vi "SyringeCalibration.vi"() -> ()   [LabVIEW 2019]
panel:
  out "ValidZ?":bool
  out "ValidY?":bool
  out "ValidX?":bool
  out "FinalXYZ":string
  in  "ExtraKaptonZ(mm)":dbl
  in  "HeightGaugeOffset(mm)":dbl=50.5
  out "CorrPosZ":dbl
  out "error out":errorcluster
  out "CorrPosY":dbl
  out "CorrPosX":dbl
  in  "BasePlatePositions":path=path "C:/Users/TTUHEP/Documents/LabVIEW/Data/AssemblyIO_logs/BaseplatePositions.txt"
  in  "RefSyringeYonTray":dbl=1216.51
  in  "RefSyringeXonTray":dbl=487.35
  in  "GHtoSyringeOffsetY":dbl=9.003
  in  "GHtoSyringeOffsetX":dbl=135.44
  in  "OnBaseplate":bool
  in  "ZcalibGcodeOnBaseplate":string="G90\nG1 Z0 F100\nG1 X368.574\tY1136.68\tF100\nG1 Z25.988 F10"
  out "TouchStatusY":bool
  out "TouchOnceY?":bool
  out "TouchStatusX":bool
  in  "StopX":bool
  out "TouchOnceX?":bool
  out "TouchedOnce?":bool
  out "TouchStatus":bool
  in  "CalibZ":bool
  in  "CalibY":bool
  in  "CalibX":bool
  out "Position Z":dbl
  in  "StopZ":bool
  out "PositionTrayY":dbl
  in  "StopY":bool
  out "PositionTrayX":dbl
  in  "milliseconds to wait":u32=500
  in  "ZcalibGcode":string="G90\nG1 Z0 F100\nG1 X290.667\tY775.823\tF100\nG1 Z36.5 F10"
  in  "YcalibGcode":string="G90\nG1 Z0 F100\nG1 X450.0 Y1217.0 F100\nG1 Z88.580 F10"
  in  "XcalibGcode":string="G90\nG1 Z0 F100\nG1 X487.5 Y1190.0 F100\nG1 Z88.580 F10"
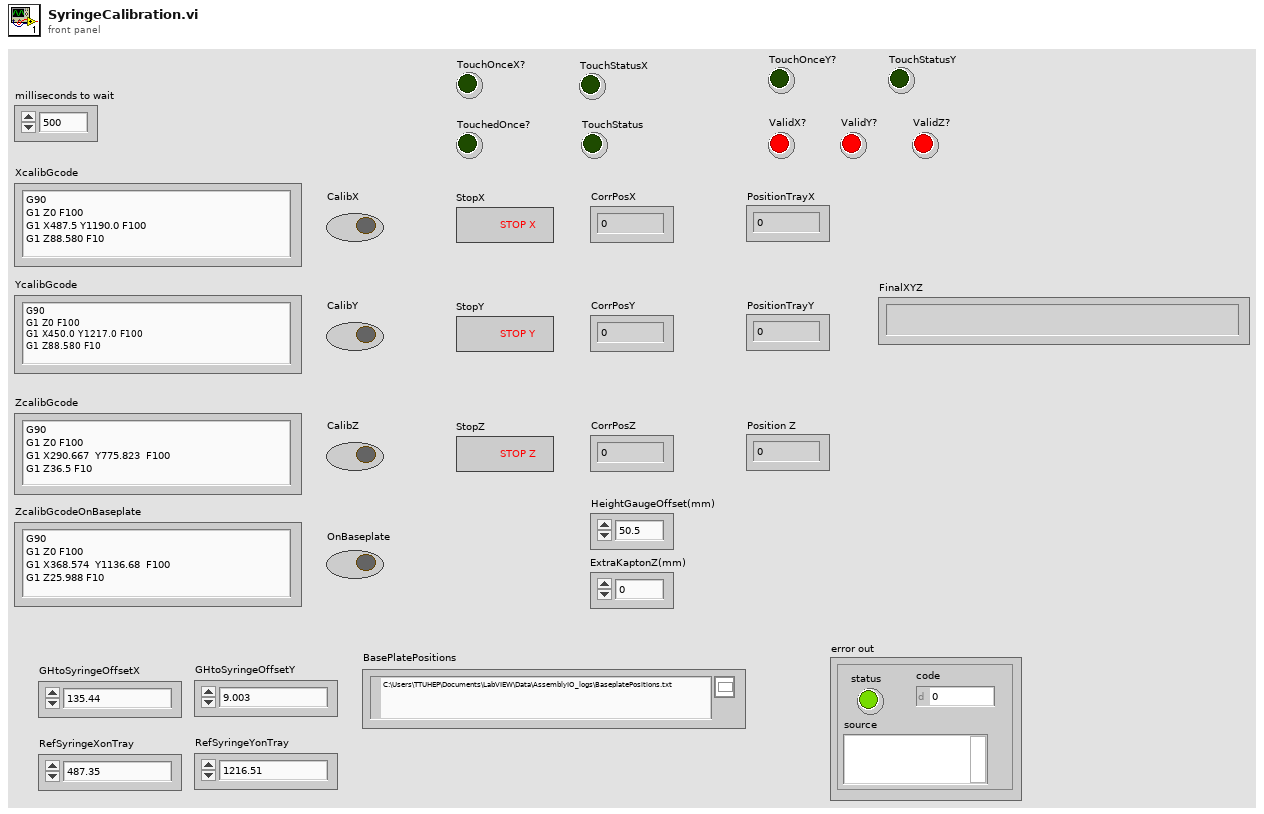
[diagram p1: front panel]
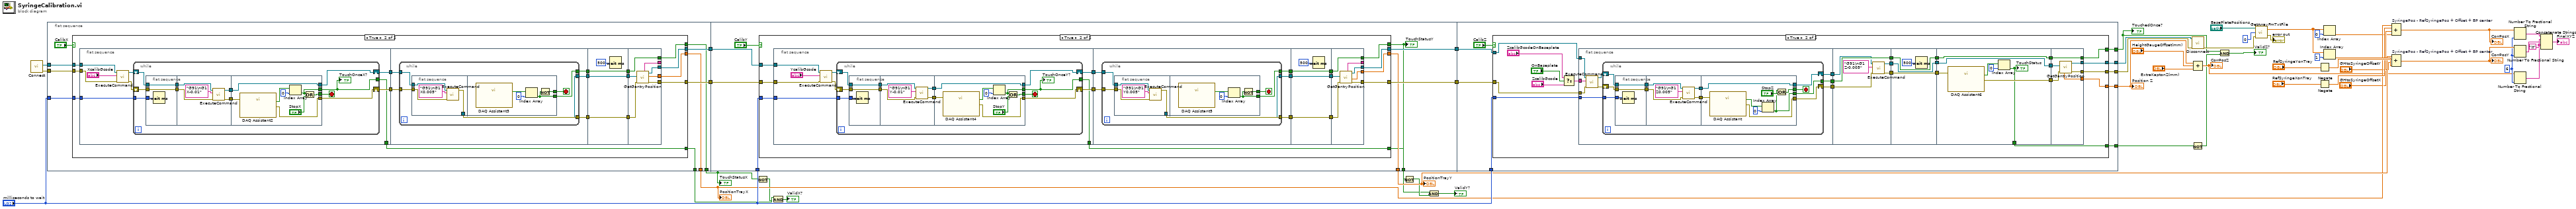
[diagram p0: block diagram]
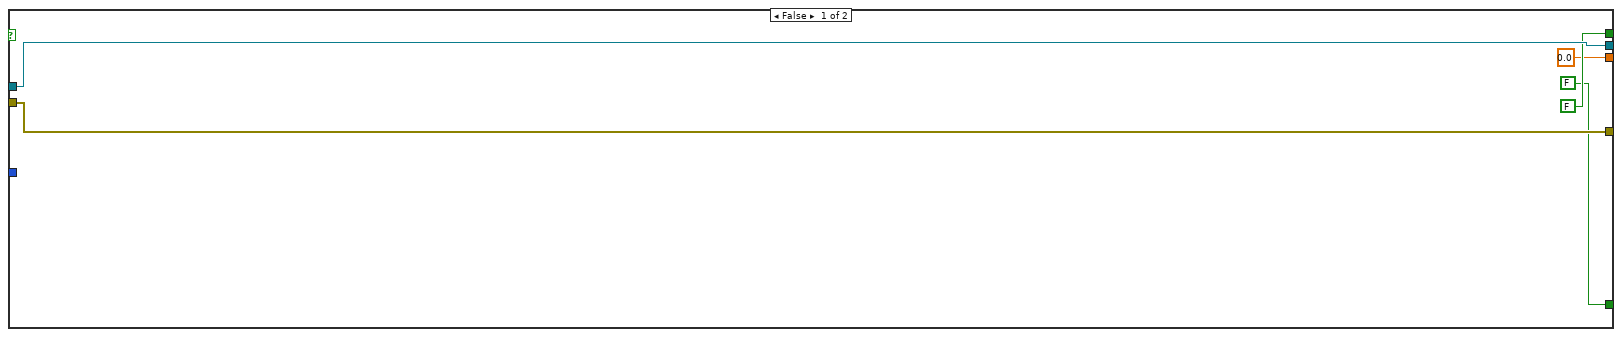
[diagram p2: hidden frame]
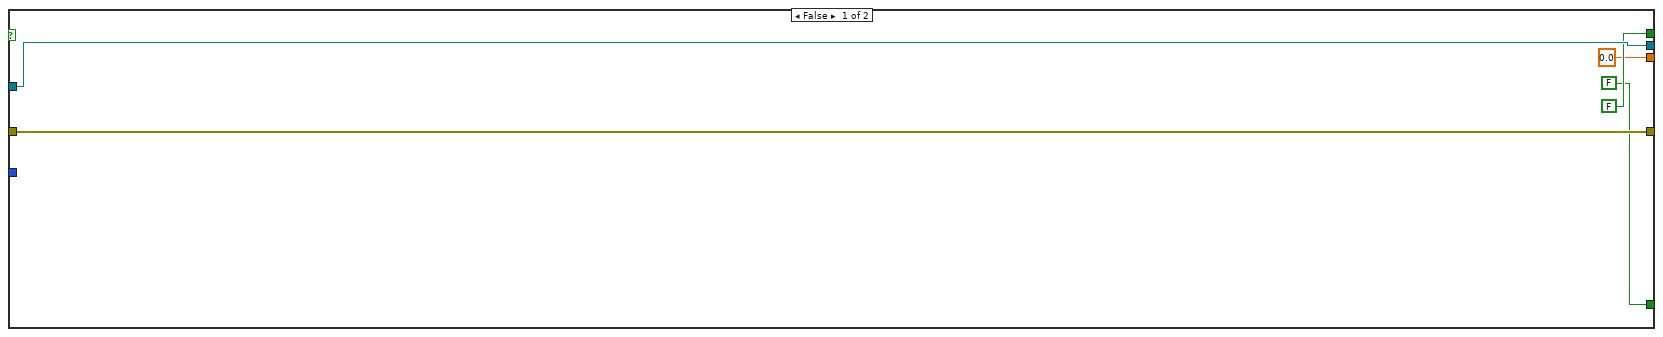
[diagram p3: hidden frame]
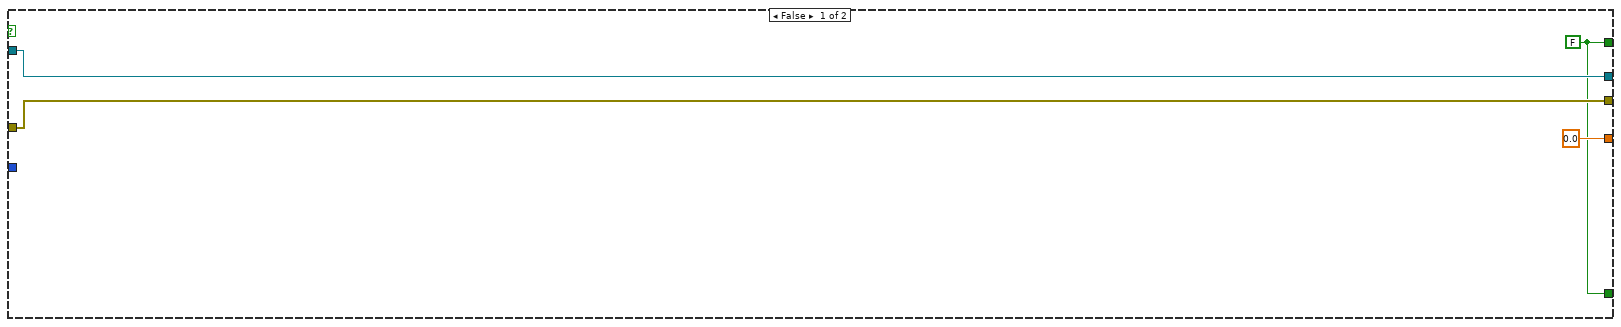
[diagram p4: hidden frame]
diagram:
  w17 = "\t"
  w19 = i16 6 ("width (-)")
  n1 = call "Connect.vi"() -> ("error out"=w47:errorcluster, "controller"=w46:refnum<k24>)  [unwired: 10 in]
  n2 = flat-sequence {
    tunnel: "milliseconds to wait" -> [w56]
    tunnel: w47 -> [w57]
    tunnel: w46 -> [w58]
    tunnel: [w55] -> w45
    tunnel: [w54] -> w44
    tunnel: [w53] -> w10
    tunnel: [w52] -> w31
    tunnel: [w51] -> w12
    tunnel: "milliseconds to wait" -> [w154]
    tunnel: w45 -> [w156]
    tunnel: w44 -> [w155]
    tunnel: [w153] -> w43
    tunnel: [w152] -> w42
    tunnel: [w150] -> w33
    tunnel: [w149] -> w6
    tunnel: [w148] -> w5
    tunnel: "milliseconds to wait" -> [w253]
    tunnel: [w252] -> w49
    tunnel: [w251] -> w48
    tunnel: w43 -> [w249]
    tunnel: [w247] -> w2
    tunnel: w42 -> [w248]
    tunnel: [w246] -> w22
    tunnel: [w245] -> w1
    frame #0 {
      n3 = case shown="True" "CalibX" {
        tunnel: w56 -> [_ w80]
        tunnel: [w64 w74] -> w54
        tunnel: [w63 w73] -> w55
        tunnel: w57 -> [w64 w78]
        tunnel: w58 -> [w63 w79]
        tunnel: [FALSE ("Boolean") w77] -> w53
        tunnel: [0.0 ("Position X") w66] -> w52
        tunnel: [FALSE ("Boolean") w65] -> w51
        frame False {
        }
        frame True {
          n4 = flat-sequence {
            tunnel: w80 -> [w89]
            tunnel: w79 -> [w86]
            tunnel: w78 -> [w85]
            tunnel: [w83] -> w76
            tunnel: [w82] -> w75
            tunnel: [w81] -> w65
            tunnel: w76 -> [w121]
            tunnel: w75 -> [w120]
            tunnel: [w117] -> w72
            tunnel: [w119] -> w70
            tunnel: [w118] -> w68
            tunnel: w72 -> [w140]
            tunnel: [w140] -> w71
            tunnel: w70 -> [w139]
            tunnel: [w139] -> w69
            tunnel: w68 -> [w138]
            tunnel: [w138] -> w67
            tunnel: [w147] -> w77
            tunnel: w71 -> [w147]
            tunnel: w69 -> [w146]
            tunnel: w67 -> [w145]
            tunnel: [w144] -> w74
            tunnel: [w143] -> w73
            tunnel: [w142] -> _
            tunnel: [w141] -> w66
            frame #0 {
              n5 = call "ExecuteCommand.vi"("error in (no error)"=w85, "Command Code"="XcalibGcode", "controller in"=w86) -> ("error out"=w88:errorcluster, "controller out"=w87:refnum<k24>)  [unwired: 6 in, 1 out]
              n6 = while {
                tunnel: w89 -> [w91]
                shift-right: [w96] -> w82
                shift-left: w87 -> [w100]
                shift-right: [w95] -> w83
                shift-left: w88 -> [w99]
                tunnel: [w90] -> w81
                stop <- w94 stop-if-true
                n7 = flat-sequence {
                  tunnel: w99 -> [w102]
                  tunnel: w100 -> [w103]
                  tunnel: [w103] -> w93
                  tunnel: [w102] -> w92
                  tunnel: w91 -> [w101]
                  tunnel: [w105] -> w98
                  tunnel: [w104] -> w97
                  tunnel: w93 -> [w107]
                  tunnel: w92 -> [w106]
                  tunnel: [w111] -> w95
                  tunnel: w98 -> [w112]
                  tunnel: [w116] -> w96
                  tunnel: w97 -> [w116]
                  tunnel: [w113] -> w94
                  tunnel: [w110] -> w90
                  frame #0 {
                    n8 = Wait (ms)(milliseconds to wait=w101) -> ()  [unwired: 1 out]
                  }
                  frame #1 {
                    n9 = call "ExecuteCommand.vi"("error in (no error)"=w106, "Command Code"="G91\nG1 X-0.01", "controller in"=w107) -> ("error out"=w105:errorcluster, "controller out"=w104:refnum<k24>)  [unwired: 6 in, 1 out]
                  }
                  frame #2 {
                    n10 = call "DAQ Assistant2"("error in"=w112) -> ("data"=w114:bool[], "error out"=w111:errorcluster)  [unwired: 16 in, 1 out]
                    n11 = Index Array(array=w114, index=0) -> (element=w110:bool)
                    n12 = Or(x=w110, y="StopX") -> (x .or. y?=w113:bool)
                  }
                }
                "TouchOnceX?" <- w90
              }
            }
            frame #1 {
              n13 = while {
                tunnel: w121 -> [w127]
                tunnel: w120 -> [w126]
                tunnel: [w125] -> w119
                tunnel: [w124] -> w118
                tunnel: [w122] -> w117
                stop <- w123 stop-if-true
                n14 = flat-sequence {
                  tunnel: w127 -> [w132]
                  tunnel: w126 -> [w130]
                  tunnel: [w129] -> w125
                  tunnel: [w128] -> w124
                  tunnel: [w134] -> w123
                  tunnel: [w133] -> w122
                  frame #0 {
                    n15 = call "ExecuteCommand.vi"("error in (no error)"=w132, "Command Code"="G91\nG1 X0.005", "controller in"=w130) -> ("error out"=w129:errorcluster, "controller out"=w128:refnum<k24>)  [unwired: 6 in, 1 out]
                  }
                  frame #1 {
                    n16 = call "DAQ Assistant3"() -> ("data"=w136:bool[])  [unwired: 17 in, 2 out]
                    n17 = Index Array(array=w136, index=0) -> (element=w133:bool)
                    n18 = Not(x=w133) -> (.not. x?=w134:bool)
                  }
                }
              }
            }
            frame #2 {
              n19 = Wait (ms)(milliseconds to wait=u32 500) -> ()  [unwired: 1 out]
            }
            frame #3 {
              n20 = call "GetGantryPosition.vi"("error in (no error)"=w146, "Controller In"=w145) -> ("error out"=w144:errorcluster, "Position X"=w141:dbl, "controller out"=w143:refnum<k24>, "Position_XYZ"=w142:string)  [unwired: 3 in, 3 out]
            }
          }
        }
      }
    }
    frame #1 {
      n21 = case shown="True" "CalibY" {
        tunnel: w154 -> [_ w177]
        tunnel: [w161 w171] -> w152
        tunnel: [w160 w170] -> w153
        tunnel: w155 -> [w161 w175]
        tunnel: w156 -> [w160 w176]
        tunnel: [FALSE ("Boolean") w174] -> w149
        tunnel: [0.0 ("Position Y") w163] -> w150
        tunnel: [FALSE ("Boolean") w162] -> w148
        frame False {
        }
        frame True {
          n22 = flat-sequence {
            tunnel: w177 -> [w186]
            tunnel: w176 -> [w183]
            tunnel: w175 -> [w182]
            tunnel: [w181] -> w173
            tunnel: [w180] -> w172
            tunnel: [w178] -> w162
            tunnel: w173 -> [w218]
            tunnel: w172 -> [w217]
            tunnel: [w214] -> w169
            tunnel: [w216] -> w167
            tunnel: [w215] -> w165
            tunnel: w169 -> [w237]
            tunnel: [w237] -> w168
            tunnel: w167 -> [w236]
            tunnel: [w236] -> w166
            tunnel: w165 -> [w235]
            tunnel: [w235] -> w164
            tunnel: [w244] -> w174
            tunnel: w168 -> [w244]
            tunnel: w166 -> [w243]
            tunnel: w164 -> [w242]
            tunnel: [w241] -> w171
            tunnel: [w240] -> w170
            tunnel: [w239] -> _
            tunnel: [w238] -> w163
            frame #0 {
              n23 = call "ExecuteCommand.vi"("error in (no error)"=w182, "Command Code"="YcalibGcode", "controller in"=w183) -> ("error out"=w185:errorcluster, "controller out"=w184:refnum<k24>)  [unwired: 6 in, 1 out]
              n24 = while {
                tunnel: w186 -> [w188]
                shift-right: [w193] -> w180
                shift-left: w184 -> [w197]
                shift-right: [w192] -> w181
                shift-left: w185 -> [w196]
                tunnel: [w187] -> w178
                stop <- w191 stop-if-true
                n25 = flat-sequence {
                  tunnel: w196 -> [w199]
                  tunnel: w197 -> [w200]
                  tunnel: [w200] -> w190
                  tunnel: [w199] -> w189
                  tunnel: w188 -> [w198]
                  tunnel: [w202] -> w195
                  tunnel: [w201] -> w194
                  tunnel: w190 -> [w204]
                  tunnel: w189 -> [w203]
                  tunnel: [w208] -> w192
                  tunnel: w195 -> [w209]
                  tunnel: [w213] -> w193
                  tunnel: w194 -> [w213]
                  tunnel: [w210] -> w191
                  tunnel: [w207] -> w187
                  frame #0 {
                    n26 = Wait (ms)(milliseconds to wait=w198) -> ()  [unwired: 1 out]
                  }
                  frame #1 {
                    n27 = call "ExecuteCommand.vi"("error in (no error)"=w203, "Command Code"="G91\nG1 Y-0.01", "controller in"=w204) -> ("error out"=w202:errorcluster, "controller out"=w201:refnum<k24>)  [unwired: 6 in, 1 out]
                  }
                  frame #2 {
                    n28 = call "DAQ Assistant4"("error in"=w209) -> ("data"=w211:bool[], "error out"=w208:errorcluster)  [unwired: 16 in, 1 out]
                    n29 = Index Array(array=w211, index=0) -> (element=w207:bool)
                    n30 = Or(x=w207, y="StopY") -> (x .or. y?=w210:bool)
                  }
                }
                "TouchOnceY?" <- w187
              }
            }
            frame #1 {
              n31 = while {
                tunnel: w218 -> [w224]
                tunnel: w217 -> [w223]
                tunnel: [w222] -> w216
                tunnel: [w221] -> w215
                tunnel: [w219] -> w214
                stop <- w220 stop-if-true
                n32 = flat-sequence {
                  tunnel: w224 -> [w229]
                  tunnel: w223 -> [w227]
                  tunnel: [w226] -> w222
                  tunnel: [w225] -> w221
                  tunnel: [w231] -> w220
                  tunnel: [w230] -> w219
                  frame #0 {
                    n33 = call "ExecuteCommand.vi"("error in (no error)"=w229, "Command Code"="G91\nG1 Y0.005", "controller in"=w227) -> ("error out"=w226:errorcluster, "controller out"=w225:refnum<k24>)  [unwired: 6 in, 1 out]
                  }
                  frame #1 {
                    n34 = call "DAQ Assistant5"() -> ("data"=w233:bool[])  [unwired: 17 in, 2 out]
                    n35 = Index Array(array=w233, index=0) -> (element=w230:bool)
                    n36 = Not(x=w230) -> (.not. x?=w231:bool)
                  }
                }
              }
            }
            frame #2 {
              n37 = Wait (ms)(milliseconds to wait=u32 500) -> ()  [unwired: 1 out]
            }
            frame #3 {
              n38 = call "GetGantryPosition.vi"("error in (no error)"=w243, "Controller In"=w242) -> ("error out"=w241:errorcluster, "Position Y"=w238:dbl, "controller out"=w240:refnum<k24>, "Position_XYZ"=w239:string)  [unwired: 3 in, 3 out]
            }
          }
        }
      }
      "TouchStatusY" <- w149
    }
    frame #2 {
      n39 = case shown="True" "CalibZ" {
        tunnel: w253 -> [_ w281]
        tunnel: [w257 w267] -> w252
        tunnel: [w256 w266] -> w251
        tunnel: w248 -> [w257 w279]
        tunnel: w249 -> [w256 w280]
        tunnel: [w254 w278] -> w247
        tunnel: [0.0 ("Position Z") w265] -> w246
        tunnel: [w254 w258] -> w245
        frame False {
          w254 = FALSE ("Boolean")
        }
        frame True {
          n40 = Select(t="ZcalibGcodeOnBaseplate", s="OnBaseplate", f="ZcalibGcode") -> (s? t:f=w274:string)
          n41 = flat-sequence {
            tunnel: w281 -> [w290]
            tunnel: w280 -> [w287]
            tunnel: w279 -> [w286]
            tunnel: w274 -> [w282]
            tunnel: [w285] -> w273
            tunnel: [w284] -> w272
            tunnel: [w283] -> w271
            tunnel: w273 -> [w323]
            tunnel: w272 -> [w322]
            tunnel: w271 -> [w321]
            tunnel: [w323] -> w270
            tunnel: [w320] -> w269
            tunnel: [w319] -> w268
            tunnel: w270 -> [w327]
            tunnel: w269 -> [w326]
            tunnel: w268 -> [w325]
            tunnel: [w327] -> w264
            tunnel: [w326] -> w262
            tunnel: [w325] -> w260
            tunnel: w264 -> [w334]
            tunnel: [w334] -> w263
            tunnel: w262 -> [w330]
            tunnel: [w329] -> w261
            tunnel: w260 -> [w333]
            tunnel: [w333] -> w259
            tunnel: [w328] -> w258
            tunnel: [w340] -> w278
            tunnel: w263 -> [w340]
            tunnel: w261 -> [w335]
            tunnel: w259 -> [w336]
            tunnel: [w339] -> w267
            tunnel: [w338] -> w266
            tunnel: [w337] -> w265
            frame #0 {
              n42 = call "ExecuteCommand.vi"("error in (no error)"=w286, "Command Code"=w282, "controller in"=w287) -> ("error out"=w289:errorcluster, "controller out"=w288:refnum<k24>)  [unwired: 6 in, 1 out]
              n43 = while {
                tunnel: w290 -> [w292]
                shift-right: [w297] -> w283
                shift-left: w288 -> [w301]
                shift-right: [w296] -> w284
                shift-left: w289 -> [w300]
                tunnel: [w291] -> w285
                stop <- w295 stop-if-true
                n44 = flat-sequence {
                  tunnel: w300 -> [w303]
                  tunnel: w301 -> [w304]
                  tunnel: [w304] -> w294
                  tunnel: [w303] -> w293
                  tunnel: w292 -> [w302]
                  tunnel: [w306] -> w299
                  tunnel: [w305] -> w298
                  tunnel: w294 -> [w308]
                  tunnel: w293 -> [w307]
                  tunnel: [w311] -> w296
                  tunnel: w299 -> [w312]
                  tunnel: [w317] -> w297
                  tunnel: w298 -> [w317]
                  tunnel: [w313] -> w295
                  tunnel: [w310] -> w291
                  frame #0 {
                    n45 = Wait (ms)(milliseconds to wait=w302) -> ()  [unwired: 1 out]
                  }
                  frame #1 {
                    n46 = call "ExecuteCommand.vi"("error in (no error)"=w307, "Command Code"="G91\nG1 Z0.005", "controller in"=w308) -> ("error out"=w306:errorcluster, "controller out"=w305:refnum<k24>)  [unwired: 6 in, 1 out]
                  }
                  frame #2 {
                    n47 = call "DAQ Assistant"("error in"=w312) -> ("data"=w314:bool[], "error out"=w311:errorcluster)  [unwired: 16 in, 1 out]
                    n48 = Index Array(array=w314, index=0) -> (element=w310:bool)
                    n49 = Or(x=w310, y="StopZ") -> (x .or. y?=w313:bool)
                  }
                }
              }
            }
            frame #1 {
              n50 = call "ExecuteCommand.vi"("error in (no error)"=w322, "Command Code"="G91\nG1 Z-0.005", "controller in"=w321) -> ("error out"=w320:errorcluster, "controller out"=w319:refnum<k24>)  [unwired: 6 in, 1 out]
            }
            frame #2 {
              n51 = Wait (ms)(milliseconds to wait=u32 500) -> ()  [unwired: 1 out]
            }
            frame #3 {
              n52 = call "DAQ Assistant6"("error in"=w330) -> ("data"=w331:bool[], "error out"=w329:errorcluster)  [unwired: 16 in, 1 out]
              n53 = Index Array(array=w331, index=0) -> (element=w328:bool)
              "TouchStatus" <- w328
            }
            frame #4 {
              n54 = call "GetGantryPosition.vi"("error in (no error)"=w335, "Controller In"=w336) -> ("error out"=w339:errorcluster, "controller out"=w338:refnum<k24>, "Position Z"=w337:dbl)  [unwired: 3 in, 4 out]
            }
          }
        }
      }
    }
  }
  n55 = Not(x=w10) -> (.not. x?=w11:bool)
  n56 = And(x=w12, y=w11) -> (x .and. y?=→"ValidX?":bool)
  n57 = Not(x=w6) -> (.not. x?=w8:bool)
  n58 = And(x=w5, y=w8) -> (x .and. y?=→"ValidY?":bool)
  n59 = Not(x=w1) -> (.not. x?=w4:bool)
  n60 = call "Disconnect.vi"("error in (no error)"=w49, "controller"=w48) -> ("error out"=w26:errorcluster)  [unwired: 9 in]
  n61 = Compound Arithmetic op=ADD(w22, "HeightGaugeOffset(mm)", "ExtraKaptonZ(mm)") -> (w18:dbl)
  "CorrPosZ" <- w18
  n62 = And(x=w2, y=w4) -> (x .and. y?=→"ValidZ?":bool)
  n63 = call "GetArrayFmTxtFile.vi"("error in"=w26, "LineNo."=0, "TextFile"="BasePlatePositions") -> ("error out"=→"error out":errorcluster, "Array"=w37:dbl[])
  n64 = Negate(x="RefSyringeYonTray") -> (-x=w35:dbl)
  n65 = Negate(x="RefSyringeXonTray") -> (-x=w32:dbl)
  n66 = Index Array(array=w37, index=0) -> (element=w27:dbl)
  n67 = Index Array(array=w37, index=1) -> (element=w34:dbl)
  n68 = Compound Arithmetic op=ADD "SyringePos - RefSyringePos + Offset + BP center"(w31, w32, "GHtoSyringeOffsetX", w27) -> (w21:dbl)
  "CorrPosX" <- w21
  n69 = Compound Arithmetic op=ADD "SyringePos - RefSyringePos + Offset + BP center"(w33, w35, "GHtoSyringeOffsetY", w34) -> (w20:dbl)
  "CorrPosY" <- w20
  n70 = Number To Fractional String(number=w21, precision (6)=w19) -> (F-format string=w16:string)  [unwired: 2 in]
  n71 = Number To Fractional String(number=w20, precision (6)=w19) -> (F-format string=w15:string)  [unwired: 2 in]
  n72 = Number To Fractional String(number=w18, precision (6)=w19) -> (F-format string=w14:string)  [unwired: 2 in]
  n73 = Concatenate Strings(w16, w17, w15, w17, w14) -> (→"FinalXYZ":string)
  "TouchedOnce?" <- w2
  "TouchStatusX" <- w10
  "PositionTrayY" <- w33
  "PositionTrayX" <- w31
  "Position Z" <- w22
